vi "Test Cycle.vi"() -> ()   [LabVIEW 2016, in "2015 VA Washer.lvlib"]
uses:
  Projects/2015 VA Washer.lvlib
  Common/LabVIEW GEA2 Toolkit/LabVIEW_GEA2_Toolkit.lvlibp/type defs/Source_Destination.ctl
  type defs/Motor Control Without Stop Start.ctl
  Common/LabVIEW GEA2 Toolkit/LabVIEW_GEA2_Toolkit.lvlibp/type defs/ERD Read Data In.ctl
  Common/LabVIEW GEA2 Toolkit/LabVIEW_GEA2_Toolkit.lvlibp/type defs/Data Type.ctl
  type defs/Drive Cycle Engine Request State.ctl
  Common/LabVIEW GEA2 Toolkit/LabVIEW_GEA2_Toolkit.lvlibp/type defs/ERD Write Data In.ctl
  Common/LabVIEW GEA2 Toolkit/LabVIEW_GEA2_Toolkit.lvlibp
panel:
  in  "Spray Rinse Time (s)":dbl=120.0 caption="Delay Time (s)"
  in  "Intermediate Spin Time":dbl=120.0 caption="Delay Time (s)"
  in  "Agitate Time (s)":dbl=30.0 caption="Delay Time (s)"
  in  "Final Spin Time (s)":dbl=180.0 format="%#_13g"
  out "Error Out":errorcluster={"status"=TRUE, "code"=1172, "source"="Invoke Node Error calling method GeaCommunication.GeaBus.Read, (System.ArgumentNullException: Key cannot be null.\r\nParameter name: key) <append><b>System.ArgumentNullException</b> in LabVIEW_GEA2_Toolkit.lvlibp:GEA2 Send and Receive Message.vi->LabVIEW_GEA2_Toolkit.lvlibp:GEA2 Write ERD.vi->Drive Cycle Engine Request State ERD.vi->Test Cycle.vi"}
  in  "Target Gallons":dbl=4.0
  in  "Error In":errorcluster
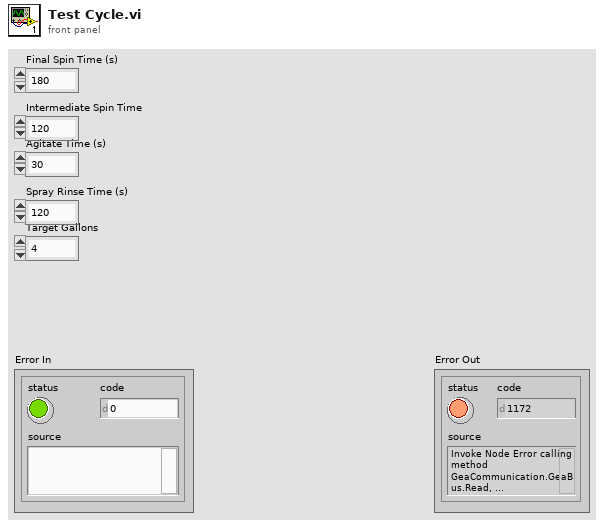
[diagram p1: front panel]
types:
  T1 = enum16{"ALL OFF", "Cold Valve", "Hot Valve", "Fabric Softener Valve", "Spray Rinse Valve", "Hot and Cold Valve"}
  T2 = typedef "LabVIEW_GEA2_Toolkit.lvlibp/ERD Write Data In.ctl" = cluster{"ERD Number":u16, "Data Type":T3, "Data":string}
  T3 = typedef "LabVIEW_GEA2_Toolkit.lvlibp/Data Type.ctl" = enum16{"string", "boolean", "uint8_t", "uint16_t", "uint32_t", "uint64_t", "int8_t", "int16_t", "int32_t", "int64_t"}
  T4 = typedef "2015 VA Washer.lvlib/Drive Cycle Engine Request State.ctl" = enum16{"Start", "Stop", "Pause", "Resume", "Select"}
  T5 = typedef "2015 VA Washer.lvlib/Motor Control Without Stop Start.ctl" = cluster{"Speed (RPM)":i16, "Motor Profile Mode":u16, "Acceleration":i16, "Angle (Degrees)":i16, "Amplitude (%)\n-CCW +CW":i16}
  T6 = enum16{"EQ (==)", "NE (!=)", "GT (>)", "LT (<)", "GE (>=)", "LE (<=)", "GTLT(> <)", "GELE (>= <=)", "GELT (>= <)", "GTLE (> <=)", "LTGT (< >)", "LEGE (<= >=)", "LEGT (<= >)", "LTGE (< >=)", "No Comparison"}
  T7 = typedef "LabVIEW_GEA2_Toolkit.lvlibp/ERD Read Data In.ctl" = cluster{"ERD Number":u16, "Data Type":T3}
  T8 = typedef "LabVIEW_GEA2_Toolkit.lvlibp/Source_Destination.ctl" = cluster{"Source":u8, "Destination":u8}
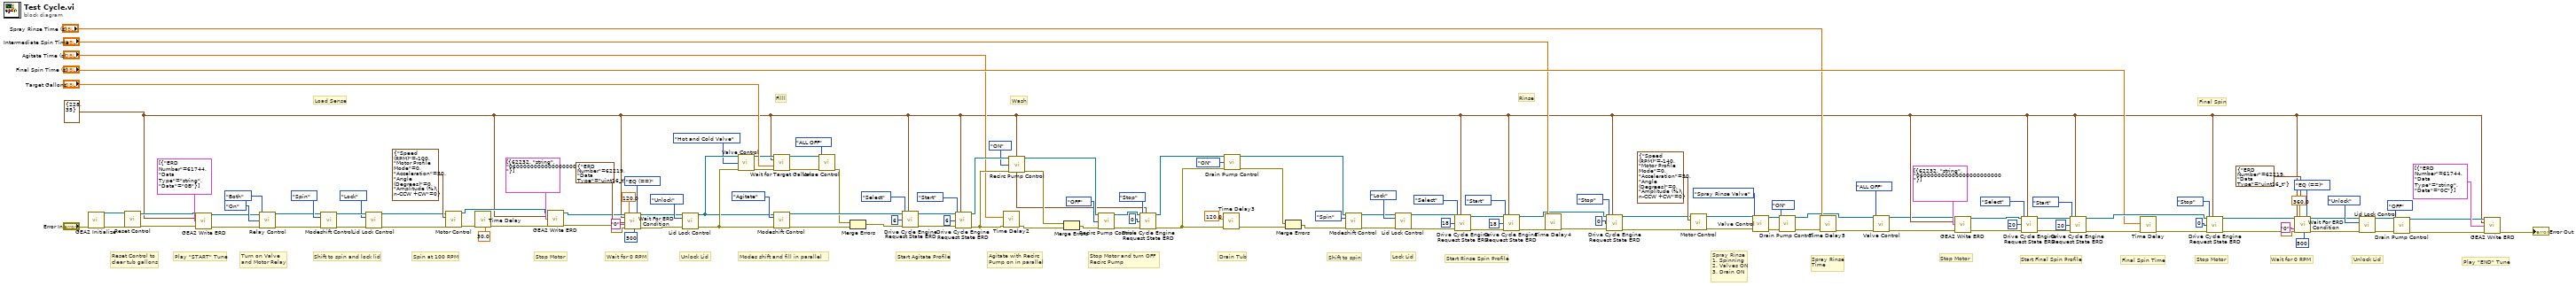
[diagram p0: block diagram]
diagram:
  w9 = T8 {"Source"=228, "Destination"=35} ("GEA Inputs")
  # "Spray Rinse\n1. Spinning\n2. Valves ON\n3. Drain ON"
  # "Spray Rinse\nTime"
  # "Stop Motor"
  # "Start Rinse Spin Profile"
  # "Load Sense"
  # "Filll"
  # "Wash"
  # "Rinse"
  # "Final Spin"
  # "Final Spin Time"
  # "Unlock Lid"
  # "Stop Motor"
  # "Lock Lid"
  # "Unlock Lid"
  # "Shift to spin"
  # "Drain Tub"
  # "Shift to spin and lock lid"
  # "Stop Motor and turn OFF \nRecirc Pump"
  # "Agitate with Recirc\nPump on in parallel"
  # "Modes shift and fill in parallel"
  # "Spin at 100 RPM"
  # "Play \"START\" Tune"
  # "Play \"END\" Tune"
  # "Reset Control to \nclear tub gallons"
  # "Stop Motor"
  # "Wait for 0 RPM"
  # "Start Final Spin Profile"
  # "Start Agitate Profile"
  # "Wait for 0 RPM"
  # "Turn on Valve \nand Motor Relay"
  n1 = call "GEA2 Initialize.vi"("error in"="Error In") -> ("GEA2 Reference Out"=w44:refnum<k24>, "error out"=w47:errorcluster)  [unwired: 12 in, 1 out]
  n2 = call "Reset Control.vi"("GEA2 Reference In"=w44, "Error In"=w47) -> ("GEA2 Reference Out"=w45:refnum<k24>, "Error Out"=w46:errorcluster)  [unwired: 10 in, 2 out]
  n3 = call "GEA2 Write ERD.vi"("GEA2 Reference In"=w45, "GEA Inputs"=w9, "Write ERD List"=T2[] [{"ERD Number"=61744, "Data Type"=enum."string", "Data"="0B"}], "Error In"=w46) -> ("GEA2 Reference Out"=w50:refnum<k24>, "Error Out"=w51:errorcluster)  [unwired: 9 in, 1 out]
  n4 = call "Relay Control.vi"("GEA2 Reference In"=w50, "Relay"=enum16{"Motor Enable", "Valve", "Both"}."Both", "State"=enum16{"On", "Off"}."On", "Error In"=w51) -> ("GEA2 Reference Out"=w131:refnum<k24>, "Error Out"=w133:errorcluster)  [unwired: 8 in, 2 out]
  n5 = call "Modeshift Control.vi"("GEA2 Reference In"=w131, "Shift To"=enum16{"Spin", "Agitate"}."Spin", "Error In"=w133) -> ("GEA2 Reference Out"=w122:refnum<k24>, "Error Out"=w123:errorcluster)  [unwired: 9 in, 2 out]
  n6 = call "Lid Lock Control.vi"("GEA2 Reference In"=w122, "Action"=enum16{"Lock", "Unlock"}."Lock", "Error In"=w123) -> ("GEA2 Reference Out"=w119:refnum<k24>, "Error Out"=w120:errorcluster)  [unwired: 9 in, 2 out]
  n7 = call "Motor Control.vi"("GEA2 Reference In"=w119, "Motor Control"=T5 {"Speed (RPM)"=-100, "Motor Profile Mode"=0, "Acceleration"=50, "Angle (Degrees)"=0, "Amplitude (%)\n-CCW +CW"=0}, "Error In"=w120) -> ("GEA2 Reference Out"=w83:refnum<k24>, "Error Out"=w128:errorcluster)  [unwired: 11 in]
  n8 = call "Time Delay"("error in (no error)"=w128, "Delay Time (s)"=30.0) -> ("error out"=w86:errorcluster)  [unwired: 9 in]
  n9 = call "GEA2 Write ERD.vi"("GEA2 Reference In"=w83, "GEA Inputs"=w9, "Write ERD List"=T2[] [{"ERD Number"=62232, "Data Type"=enum."string", "Data"="060000000000000000000000"}], "Error In"=w86) -> ("GEA2 Reference Out"=w82:refnum<k24>, "Error Out"=w85:errorcluster)  [unwired: 9 in, 1 out]
  n10 = call "Wait For ERD Condition.vi"("GEA2 Reference In"=w82, "GEA Inputs"=w9, "ERD Read Data"=T7 {"ERD Number"=62219, "Data Type"=enum."uint16_t"}, "Expected Low"="0", "Error In"=w85, "Timeout (s)"=120.0, "Loop Rate (ms)"=u32 500, "Comparison"=T6."EQ (==)") -> ("GEA2 Reference Out"=w116:refnum<k24>, "Error Out"=w118:errorcluster)  [unwired: 7 in, 3 out]
  n11 = call "Lid Lock Control.vi"("GEA2 Reference In"=w116, "Action"=enum16{"Lock", "Unlock"}."Unlock", "Error In"=w118) -> ("GEA2 Reference Out"=w93:refnum<k24>, "Error Out"=w115:errorcluster)  [unwired: 9 in, 2 out]
  n12 = call "Valve Control.vi"("GEA2 Reference In"=w93, "Fixed  Valve Control"=T1."Hot and Cold Valve", "Error In"=w115) -> ("GEA2 Reference Out"=w138:refnum<k24>, "Error Out"=w139:errorcluster)  [unwired: 11 in]
  n13 = call "Modeshift Control.vi"("GEA2 Reference In"=w93, "Shift To"=enum16{"Spin", "Agitate"}."Agitate", "Error In"=w115) -> ("GEA2 Reference Out"=w114:refnum<k24>, "Error Out"=w107:errorcluster)  [unwired: 9 in, 2 out]
  n14 = call "Wait for Target Gallons.vi"(".NET Refnum in"=w138, "GEA Inputs"=w9, "Target Gallons"="Target Gallons", "error in (no error)"=w139) -> ("GEA2 Reference Out"=w136:refnum<k24>, "error out"=w137:errorcluster)  [unwired: 10 in]
  n15 = call "Valve Control.vi"("GEA2 Reference In"=w136, "Fixed  Valve Control"=T1."ALL OFF", "Error In"=w137) -> ("Error Out"=w105:errorcluster)  [unwired: 11 in, 1 out]
  n16 = Merge Errors(w105, w107) -> (w106:errorcluster)
  n17 = call "Drive Cycle Engine Request State ERD.vi"("GEA2 Reference In"=w114, "GEA Inputs"=w9, "Cycle ID"=u8 6, "Drive Cycle Engine Request State"=Drive_Cycle_Engine_Request_State."Select", "Error In"=w106) -> ("GEA2 Reference Out"=w109:refnum<k24>, "Error Out"=w108:errorcluster)  [unwired: 9 in]
  n18 = call "Drive Cycle Engine Request State ERD.vi"("GEA2 Reference In"=w109, "GEA Inputs"=w9, "Cycle ID"=u8 6, "Drive Cycle Engine Request State"=Drive_Cycle_Engine_Request_State."Start", "Error In"=w108) -> ("GEA2 Reference Out"=w79:refnum<k24>, "Error Out"=w80:errorcluster)  [unwired: 9 in]
  n19 = call "Time Delay2"("error in (no error)"=w80, "Delay Time (s)"="Agitate Time (s)") -> ("error out"=w77:errorcluster)  [unwired: 9 in]
  n20 = call "Recirc Pump Control.vi"("GEA2 Reference In"=w79, "Drain Pump State"=enum16{"OFF", "ON"}."ON", "Error In"=w80) -> ("GEA2 Reference Out"=w73:refnum<k24>, "Error Out"=w76:errorcluster)  [unwired: 11 in]
  n21 = Merge Errors(w76, w77) -> (w75:errorcluster)
  n22 = call "Recirc Pump Control.vi"("GEA2 Reference In"=w73, "Drain Pump State"=enum16{"OFF", "ON"}."OFF", "Error In"=w75) -> ("GEA2 Reference Out"=w60:refnum<k24>, "Error Out"=w62:errorcluster)  [unwired: 11 in]
  n23 = call "Drive Cycle Engine Request State ERD.vi"("GEA2 Reference In"=w60, "GEA Inputs"=w9, "Cycle ID"=u8 0, "Drive Cycle Engine Request State"=Drive_Cycle_Engine_Request_State."Stop", "Error In"=w62) -> ("GEA2 Reference Out"=w59:refnum<k24>, "Error Out"=w61:errorcluster)  [unwired: 9 in]
  n24 = call "Time Delay3"("error in (no error)"=w61, "Delay Time (s)"=120.0) -> ("error out"=w71:errorcluster)  [unwired: 9 in]
  n25 = call "Drain Pump Control.vi"("GEA2 Reference In"=w59, "Drain Pump State"=enum16{"OFF", "ON"}."ON", "Error In"=w61) -> ("GEA2 Reference Out"=w67:refnum<k24>, "Error Out"=w70:errorcluster)  [unwired: 11 in]
  n26 = Merge Errors(w70, w71) -> (w68:errorcluster)
  n27 = call "Modeshift Control.vi"("GEA2 Reference In"=w67, "Shift To"=enum16{"Spin", "Agitate"}."Spin", "Error In"=w68) -> ("GEA2 Reference Out"=w90:refnum<k24>, "Error Out"=w92:errorcluster)  [unwired: 9 in, 2 out]
  n28 = call "Lid Lock Control.vi"("GEA2 Reference In"=w90, "Action"=enum16{"Lock", "Unlock"}."Lock", "Error In"=w92) -> ("GEA2 Reference Out"=w31:refnum<k24>, "Error Out"=w35:errorcluster)  [unwired: 9 in, 2 out]
  n29 = call "Drive Cycle Engine Request State ERD.vi"("GEA2 Reference In"=w31, "GEA Inputs"=w9, "Cycle ID"=u8 18, "Drive Cycle Engine Request State"=Drive_Cycle_Engine_Request_State."Select", "Error In"=w35) -> ("GEA2 Reference Out"=w37:refnum<k24>, "Error Out"=w36:errorcluster)  [unwired: 9 in]
  n30 = call "Drive Cycle Engine Request State ERD.vi"("GEA2 Reference In"=w37, "GEA Inputs"=w9, "Cycle ID"=u8 18, "Drive Cycle Engine Request State"=Drive_Cycle_Engine_Request_State."Start", "Error In"=w36) -> ("GEA2 Reference Out"=w19:refnum<k24>, "Error Out"=w33:errorcluster)  [unwired: 9 in]
  n31 = call "Time Delay4"("error in (no error)"=w33, "Delay Time (s)"="Intermediate Spin Time") -> ("error out"=w22:errorcluster)  [unwired: 9 in]
  n32 = call "Drive Cycle Engine Request State ERD.vi"("GEA2 Reference In"=w19, "GEA Inputs"=w9, "Cycle ID"=u8 0, "Drive Cycle Engine Request State"=Drive_Cycle_Engine_Request_State."Stop", "Error In"=w22) -> ("GEA2 Reference Out"=w11:refnum<k24>, "Error Out"=w21:errorcluster)  [unwired: 9 in]
  n33 = call "Motor Control.vi"("GEA2 Reference In"=w11, "Motor Control"=T5 {"Speed (RPM)"=-140, "Motor Profile Mode"=0, "Acceleration"=50, "Angle (Degrees)"=0, "Amplitude (%)\n-CCW +CW"=0}, "Error In"=w21) -> ("GEA2 Reference Out"=w29:refnum<k24>, "Error Out"=w30:errorcluster)  [unwired: 11 in]
  n34 = call "Valve Control.vi"("GEA2 Reference In"=w29, "Fixed  Valve Control"=T1."Spray Rinse Valve", "Error In"=w30) -> ("GEA2 Reference Out"=w27:refnum<k24>, "Error Out"=w28:errorcluster)  [unwired: 11 in]
  n35 = call "Drain Pump Control.vi"("GEA2 Reference In"=w27, "Drain Pump State"=enum16{"OFF", "ON"}."ON", "Error In"=w28) -> ("GEA2 Reference Out"=w5:refnum<k24>, "Error Out"=w25:errorcluster)  [unwired: 11 in]
  n36 = call "Time Delay5"("error in (no error)"=w25, "Delay Time (s)"="Spray Rinse Time (s)") -> ("error out"=w8:errorcluster)  [unwired: 9 in]
  n37 = call "Valve Control.vi"("GEA2 Reference In"=w5, "Fixed  Valve Control"=T1."ALL OFF", "Error In"=w8) -> ("GEA2 Reference Out"=w6:refnum<k24>, "Error Out"=w7:errorcluster)  [unwired: 11 in]
  n38 = call "GEA2 Write ERD.vi"("GEA2 Reference In"=w6, "GEA Inputs"=w9, "Write ERD List"=T2[] [{"ERD Number"=62232, "Data Type"=enum."string", "Data"="060000000000000000000000"}], "Error In"=w7) -> ("GEA2 Reference Out"=w12:refnum<k24>, "Error Out"=w17:errorcluster)  [unwired: 9 in, 1 out]
  n39 = call "Drive Cycle Engine Request State ERD.vi"("GEA2 Reference In"=w12, "GEA Inputs"=w9, "Cycle ID"=u8 20, "Drive Cycle Engine Request State"=Drive_Cycle_Engine_Request_State."Select", "Error In"=w17) -> ("GEA2 Reference Out"=w102:refnum<k24>, "Error Out"=w103:errorcluster)  [unwired: 9 in]
  n40 = call "Drive Cycle Engine Request State ERD.vi"("GEA2 Reference In"=w102, "GEA Inputs"=w9, "Cycle ID"=u8 20, "Drive Cycle Engine Request State"=Drive_Cycle_Engine_Request_State."Start", "Error In"=w103) -> ("GEA2 Reference Out"=w81:refnum<k24>, "Error Out"=w65:errorcluster)  [unwired: 9 in]
  n41 = call "Time Delay"("error in (no error)"=w65, "Delay Time (s)"="Final Spin Time (s)") -> ("error out"=w43:errorcluster)  [unwired: 9 in]
  n42 = call "Drive Cycle Engine Request State ERD.vi"("GEA2 Reference In"=w81, "GEA Inputs"=w9, "Cycle ID"=u8 0, "Drive Cycle Engine Request State"=Drive_Cycle_Engine_Request_State."Stop", "Error In"=w43) -> ("GEA2 Reference Out"=w56:refnum<k24>, "Error Out"=w55:errorcluster)  [unwired: 9 in]
  n43 = call "Wait For ERD Condition.vi"("GEA2 Reference In"=w56, "GEA Inputs"=w9, "ERD Read Data"=T7 {"ERD Number"=62219, "Data Type"=enum."uint16_t"}, "Expected Low"="0", "Error In"=w55, "Timeout (s)"=360.0, "Loop Rate (ms)"=u32 500, "Comparison"=T6."EQ (==)") -> ("GEA2 Reference Out"=w87:refnum<k24>, "Error Out"=w88:errorcluster)  [unwired: 7 in, 3 out]
  n44 = call "Lid Lock Control.vi"("GEA2 Reference In"=w87, "Action"=enum16{"Lock", "Unlock"}."Unlock", "Error In"=w88) -> ("GEA2 Reference Out"=w14:refnum<k24>, "Error Out"=w16:errorcluster)  [unwired: 9 in, 2 out]
  n45 = call "Drain Pump Control.vi"("GEA2 Reference In"=w14, "Drain Pump State"=enum16{"OFF", "ON"}."OFF", "Error In"=w16) -> ("GEA2 Reference Out"=w13:refnum<k24>, "Error Out"=w15:errorcluster)  [unwired: 11 in]
  n46 = call "GEA2 Write ERD.vi"("GEA2 Reference In"=w13, "GEA Inputs"=w9, "Write ERD List"=T2[] [{"ERD Number"=61744, "Data Type"=enum."string", "Data"="0C"}], "Error In"=w15) -> ("Error Out"=→"Error Out":errorcluster)  [unwired: 9 in, 2 out]
